vi "WSVCAP SHL Host TL SPI_RFFE Query Cycle Count.vi"(11 "error in":errorcluster, 14 "FPGA":T1) -> (4 "Cycle Count":u64, 15 "error out":errorcluster)   [LabVIEW 2017]
uses:
  Type Defs/WSVCAP SHL FPGA Enum.ctl
  Type Defs/WSVCAP SHL Top Level Control Operation Enum.ctl
  Type Defs/WSVCAP SHL Top Level Control Enum.ctl
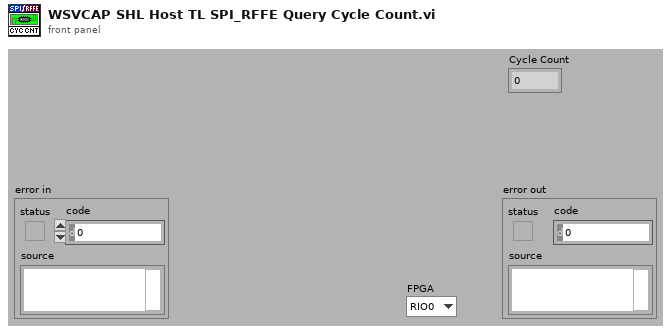
[diagram p1: front panel]
types:
  T1 = typedef "WSVCAP SHL FPGA Enum.ctl" = enum16{"RIO0", "RIO1"}
  T2 = typedef "WSVCAP SHL Top Level Control Enum.ctl" = enum16{"Start", "Cmd", "Transaction", "Wait Ticks", "Socket Mask", "UUT Set", "Slave Address", "Sub Address", "Bytes to Write", "Bytes to Read", "Write Data", "Write Flag", "Read Data", "Read Flag", "Ack Read", "Read Status Flag", "Ack Read Status", "Status", "Cycle Count", "Stop Cycle", "Exit"}
  T3 = typedef "WSVCAP SHL Top Level Control Operation Enum.ctl" = enum16{"Initialize", "Set Control", "Read Control", "Close"}
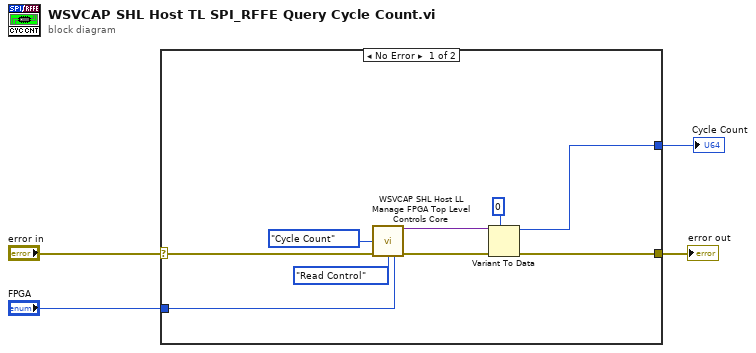
[diagram p0: block diagram]
diagram:
  n1 = case shown="No Error" "error in" {
    selector: "error in" -> [w11 _]
    tunnel: [w9 _] -> w4
    tunnel: [w6 _] -> w2
    tunnel: "FPGA" -> [w5 _]
    frame No Error {
      n2 = call "WSVCAP SHL Host LL Manage FPGA Top Level Controls Core.vi"("FPGA Top Level Control"=WSVCAP_SHL_Top_Level_Control_Enum."Cycle Count", "error in (no error)"=w11, "Operation"=WSVCAP_SHL_Top_Level_Control_Operation_Enum."Read Control", "FPGA"=w5) -> ("Value Out"=w8:variant, "error out"=w10:errorcluster)  [unwired: 10 in]
      n3 = Variant To Data(error in=w10, type=u64 0, Variant=w8) -> (data=w6:u64, error out=w9:errorcluster)
    }
    frame Error {
    }
  }
  "error out" <- w4
  "Cycle Count" <- w2
